vi "Express VI - Relay.vi"() -> ()   [LabVIEW 2023]
doc: "This example shows how to switch a signal on and off using the relay Express VI."
uses:
  Instance           1 20Saved   Relay Switch .vi
  Instance           2 20Saved   Relay Switch .vi
  Instance           4 20Saved   Relay Switch .vi
  Instance           5 20Saved   Relay Switch .vi
  Instance           3 20Saved   Relay Switch .vi
panel:
  out "Waveform Chart 1":dynamicdata(graph)
  in  "Enable":bool
  in  "Stop":bool
  out "Waveform Chart 2":dynamicdata(graph)
  # "Overview: Demonstrates how to switch a signal on and off using the Relay Express VI.\nInstructions:\n1. Run the VI.\n2. Click the Enable button. When it is set to true, the input signals will be passed to the output chart.\n3. Click Stop to stop the VI."
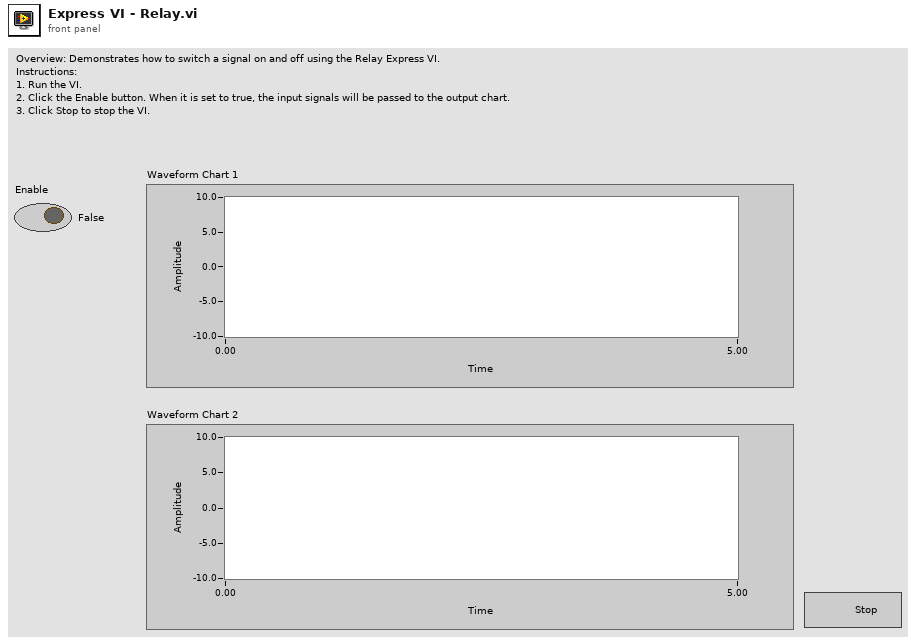
[diagram p1: front panel]
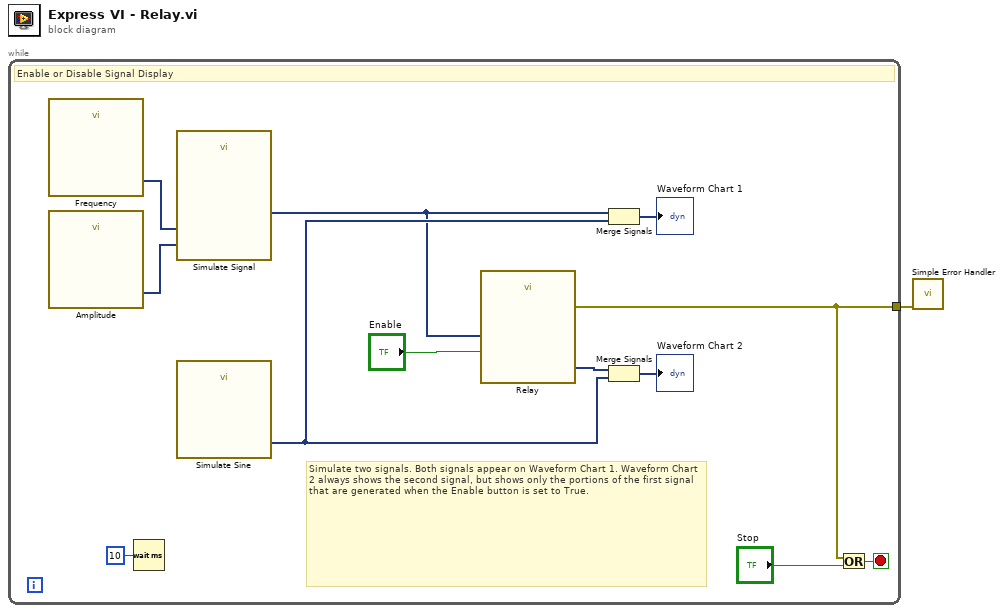
[diagram p0: block diagram]
diagram:
  n1 = while {
    tunnel: [w2] -> w1
    stop <- w3 stop-if-true
    # "Simulate two signals. Both signals appear on Waveform Chart 1. Waveform Chart 2 always shows the second signal, but shows only the portions of the first signal that are generated when the Enable button is set to True."
    # "Enable or Disable Signal Display"
    n2 = call "Frequency"() -> ("Sine"=w9:dynamicdata)  [unwired: 14 in, 1 out]
    n3 = call "Amplitude"() -> ("Sine"=w8:dynamicdata)  [unwired: 14 in, 1 out]
    n4 = Wait (ms)(milliseconds to wait=u32 10) -> ()  [unwired: 1 out]
    n5 = call "Simulate Signal"("Frequency"=w9, "Amplitude"=w8) -> ("Sine"=w7:dynamicdata)  [unwired: 12 in, 1 out]
    n6 = call "Simulate Sine"() -> ("Sine"=w10:dynamicdata)  [unwired: 14 in, 1 out]
    n7 = call "Relay"("Enable"="Enable", "Signals"=w7) -> ("error out"=w2:errorcluster, "Result"=w5:dynamicdata)  [unwired: 8 in]
    n8 = Merge Signals(w7, w10) -> (→"Waveform Chart 1":dynamicdata)
    n9 = Merge Signals(w5, w10) -> (→"Waveform Chart 2":dynamicdata)
    n10 = Or(x=w2, y="Stop") -> (x .or. y?=w3:bool)
  }
  n11 = call <vilib>:"Simple Error Handler.vi"("error in (no error)"=w1) -> ()  [unwired: 4 in, 5 out]
